vi "SQL_创建数据库.vi"(7 "数据库名称":string, 8 "error in (no error)":errorcluster, 9 "事务日志文件":T1, 10 "主数据文件":T1, 11 "connection reference":T2) -> (0 "error out":errorcluster)   [LabVIEW 2014]
uses:
  <vilib>/addons/database/Connection.llb/Conn ObjectReference.ctl
  <vilib>/addons/database/Connection.llb/Conn Execute.vi
  <vilib>/addons/database/Recordset.llb/Rec Destroy - Connection.vi
  <vilib>/addons/database/NI_Database_API.lvlib
panel:
  # "例: 3MB"
  # "例: 100MB"
  # "例: 10%"
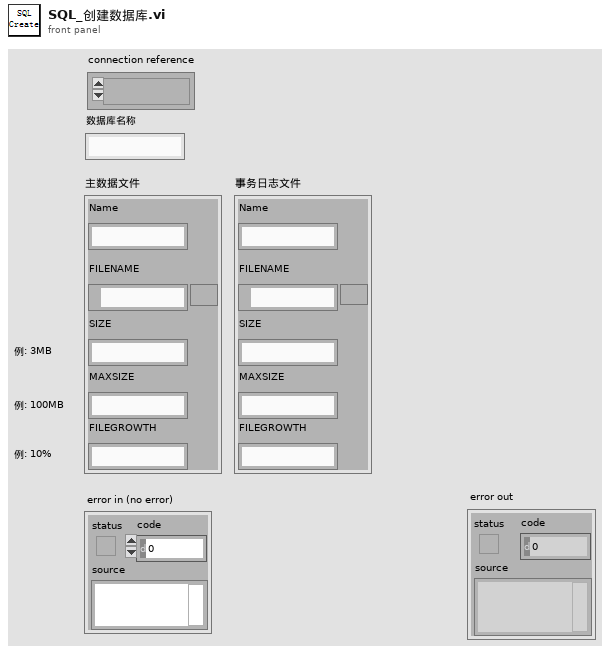
[diagram p1: front panel]
types:
  T1 = cluster{"Name":string, "FILENAME":path, "SIZE":string, "MAXSIZE":string, "FILEGROWTH":string}
  T2 = typedef "NI_Database_API.lvlib/Conn ObjectReference.ctl" = refnum<k1>
  T3 = typedef "NI_Database_API.lvlib/Rec ObjectReference.ctl" = refnum<k1>
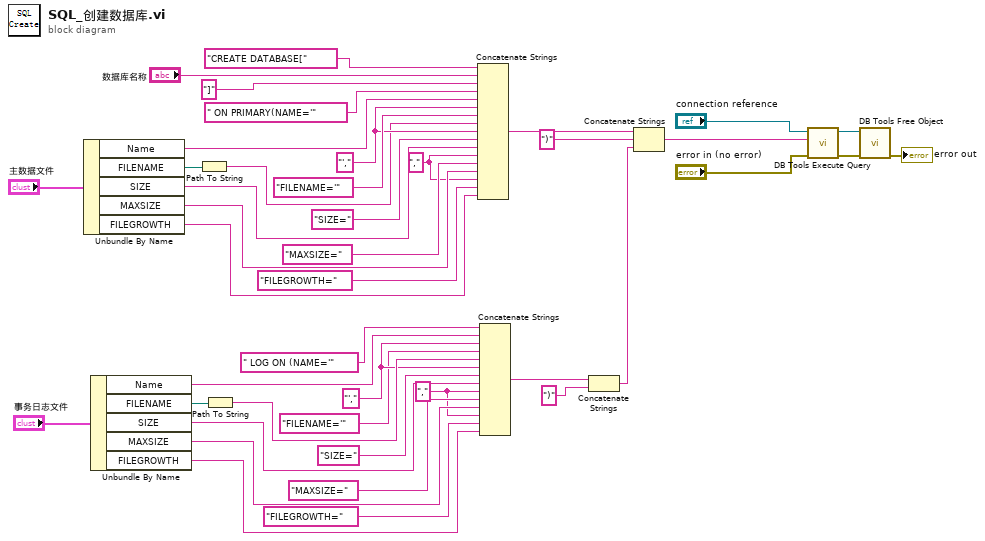
[diagram p0: block diagram]
diagram:
  w4 = "," ("字符串")
  w11 = "," ("字符串")
  w27 = "'," ("字符串")
  w34 = "'," ("字符串")
  n1 = Unbundle By Name("主数据文件") -> ("Name"=w38:string, "FILENAME"=w32:path, "SIZE"=w35:string, "MAXSIZE"=w12:string, "FILEGROWTH"=w9:string)
  n2 = Unbundle By Name("事务日志文件") -> ("Name"=w24:string, "FILENAME"=w29:path, "SIZE"=w7:string, "MAXSIZE"=w5:string, "FILEGROWTH"=w2:string)
  n3 = Path To String(path=w32) -> (string=w31:string)
  n4 = Path To String(path=w29) -> (string=w30:string)
  n5 = Concatenate Strings("CREATE DATABASE[", "数据库名称", "]" ("字符串"), " ON PRIMARY(NAME='" ("字符串"), w38, w34, "FILENAME='" ("字符串"), w31, w34, "SIZE=" ("字符串"), w35, w11, "MAXSIZE=" ("字符串"), w12, w11, "FILEGROWTH=" ("字符串"), w9) -> (w8:string)
  n6 = Concatenate Strings(" LOG ON (NAME='" ("字符串"), w24, w27, "FILENAME='" ("字符串"), w30, w27, "SIZE=" ("字符串"), w7, w4, "MAXSIZE=" ("字符串"), w5, w4, "FILEGROWTH=" ("字符串"), w2) -> (w1:string)
  n7 = Concatenate Strings(w1, ")" ("字符串")) -> (w20:string)
  n8 = Concatenate Strings(w8, ")" ("字符串"), w20) -> (w14:string)
  n9 = call-poly <vilib>:"DB Tools Execute Query.vi"("error in (no error)"="error in (no error)", "SQL query"=w14, "connection reference"="connection reference") -> ("error out"=w15:errorcluster, "recordset reference"=w16:T3)  [unwired: 5 in]
  n10 = call-poly <vilib>:"DB Tools Free Object.vi"("error in (no error)"=w15, "recordset reference"=w16) -> ("error out"=→"error out":errorcluster)  [unwired: 8 in, 1 out]
